vi "Identities.vi"(8 "error in (no error)":errorcluster, 11 "DataHandlerAPI in":refnum<class "DataHandlerAPI.lvclass">) -> (0 "error out":errorcluster, 2 "Identities":refnum<class "Identity.lvclass">[](array[class]), 3 "DataHandlerAPI out":refnum<class "DataHandlerAPI.lvclass">)   [LabVIEW 2020, in "Volatus.lvlib" / "DataHandlerAPI.lvclass"]
uses:
  DataHandlerAPI.lvclass
  DataHandlerAPI.lvclass/DataHandlerAPI.ctl
  DataHandlerIdentity/DataHandlerIdentity.lvclass
  C:/dev/lv20CE/relink/lv-volatus/Volatus/DataHandlerIdentity/DataHandlerIdentity.lvclass
  C:/dev/lv20CE/relink/lv-volatus/Volatus/Identity/Identity.lvclass
  Identity/Identity.lvclass
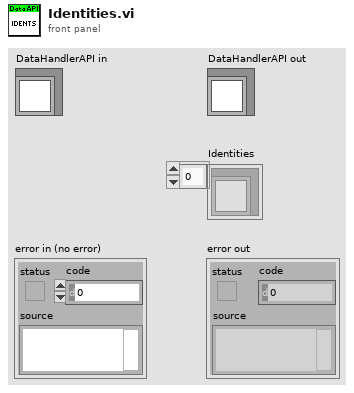
[diagram p1: front panel]
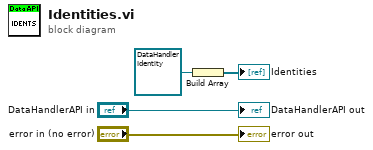
[diagram p0: block diagram]
diagram:
  n1 = Build Array(refnum<class "DataHandlerIdentity.lvclass"> refnum ("Volatus:DataHandlerIdentity.lvclass")) -> (→"Identities":refnum<class "DataHandlerIdentity.lvclass">[])
  "error out" <- "error in (no error)"
  "DataHandlerAPI out" <- "DataHandlerAPI in"
